vi "SDPC - Pause Transfer.vi"(3 "error in (no error)":errorcluster, 4 "RD/nWR":bool, 5 "Pause transfer":bool) -> (0 "error out":errorcluster, 2 "Transfer paused":bool)   [LabVIEW 2020]
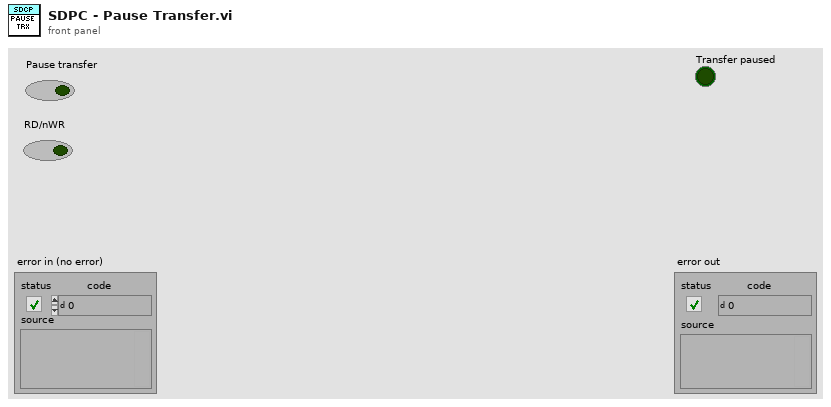
[diagram p1: front panel]
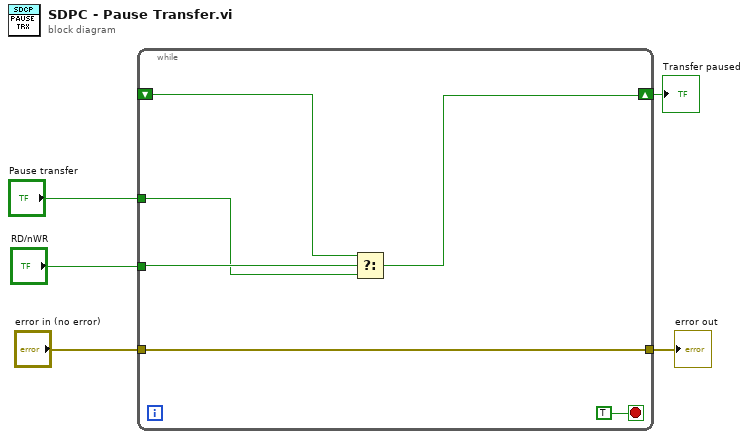
[diagram p0: block diagram]
diagram:
  n1 = while {
    shift-right: [w7] -> w1
    shift-left: _ -> [w6]
    tunnel: "error in (no error)" -> [w10]
    tunnel: [w10] -> w4
    tunnel: "Pause transfer" -> [w8]
    tunnel: "RD/nWR" -> [w9]
    stop <- TRUE stop-if-true
    n2 = Select(t=w6, s=w9, f=w8) -> (s? t:f=w7:bool)
  }
  "error out" <- w4
  "Transfer paused" <- w1
